vi "Close Interlock.vi"(8 "error in (no error)":errorcluster, 11 "Interlock in":refnum<class "Interlock.lvclass">) -> (0 "error out":errorcluster, 3 "Interlock out":refnum<class "Interlock.lvclass">)   [LabVIEW 2015, in "Interlocks.lvlib" / "Interlock.lvclass"]
uses:
  Interlock.lvclass
  Interlock.lvclass/Interlock.ctl
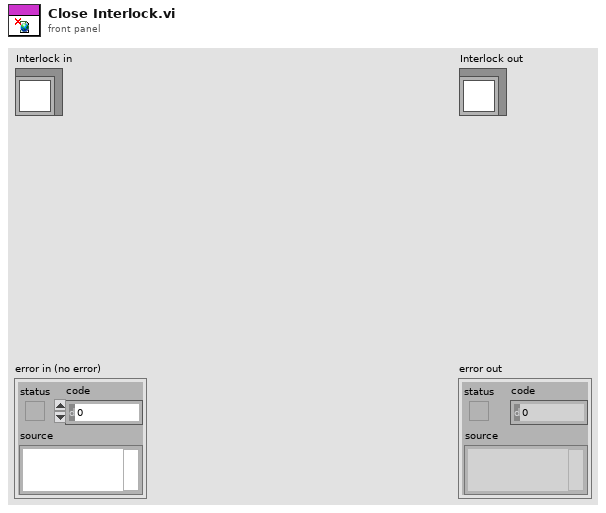
[diagram p1: front panel]
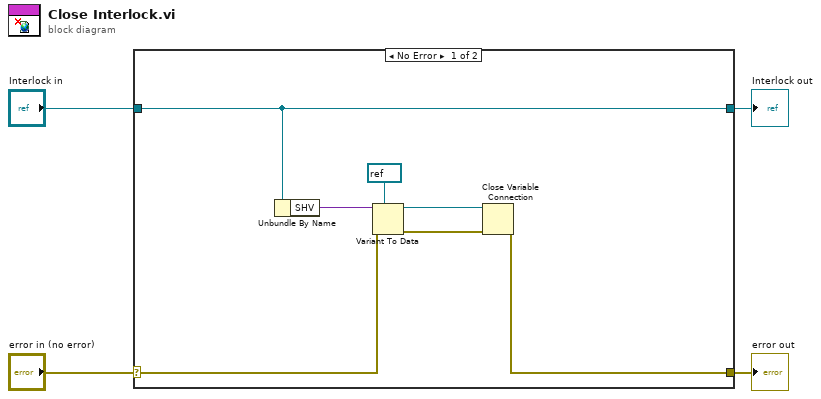
[diagram p0: block diagram]
diagram:
  n1 = case shown="No Error" "error in (no error)" {
    selector: "error in (no error)" -> [w7 w13]
    tunnel: [w9 w13] -> w3
    tunnel: [w11 w12] -> w1
    tunnel: "Interlock in" -> [w11 w12]
    frame No Error {
      n2 = Unbundle By Name(w11) -> ("SHV"=w10:variant)
      n3 = Variant To Data(error in=w7, type=refnum<k21> refnum ("SHV"), Variant=w10) -> (data=w5:refnum<k21>, error out=w6:errorcluster)
      n4 = Close Variable Connection(8:w6, 11:w5) -> (0:w9:errorcluster)
    }
    frame Error {
    }
  }
  "error out" <- w3
  "Interlock out" <- w1
